vi "Vision Processing.vi"(4 "error in (no error)":errorcluster, 7 "Image Size":T1=enum."320x240") -> ()   [LabVIEW 2018]
doc: "This VI runs in parallel to other tasks. It gets images from the camera, processes them for color or shape and use that information to affect robot behavior."
uses:
  <vilib>/Rock Robotics/WPI/Camera/WPI_CameraImageSize.ctl
  <vilib>/Rock Robotics/WPI/Camera/WPI_CameraWhite Balance Values.ctl
  <vilib>/Rock Robotics/WPI/Camera/WPI_CameraExposure Values.ctl
  <vilib>/Rock Robotics/WPI/Camera/WPI_CameraFrameRate.ctl
  Robot Global Data.vi
panel:
  in  "Image Size 2":T1=enum."320x240"
  in  "error in (no error) 2":errorcluster
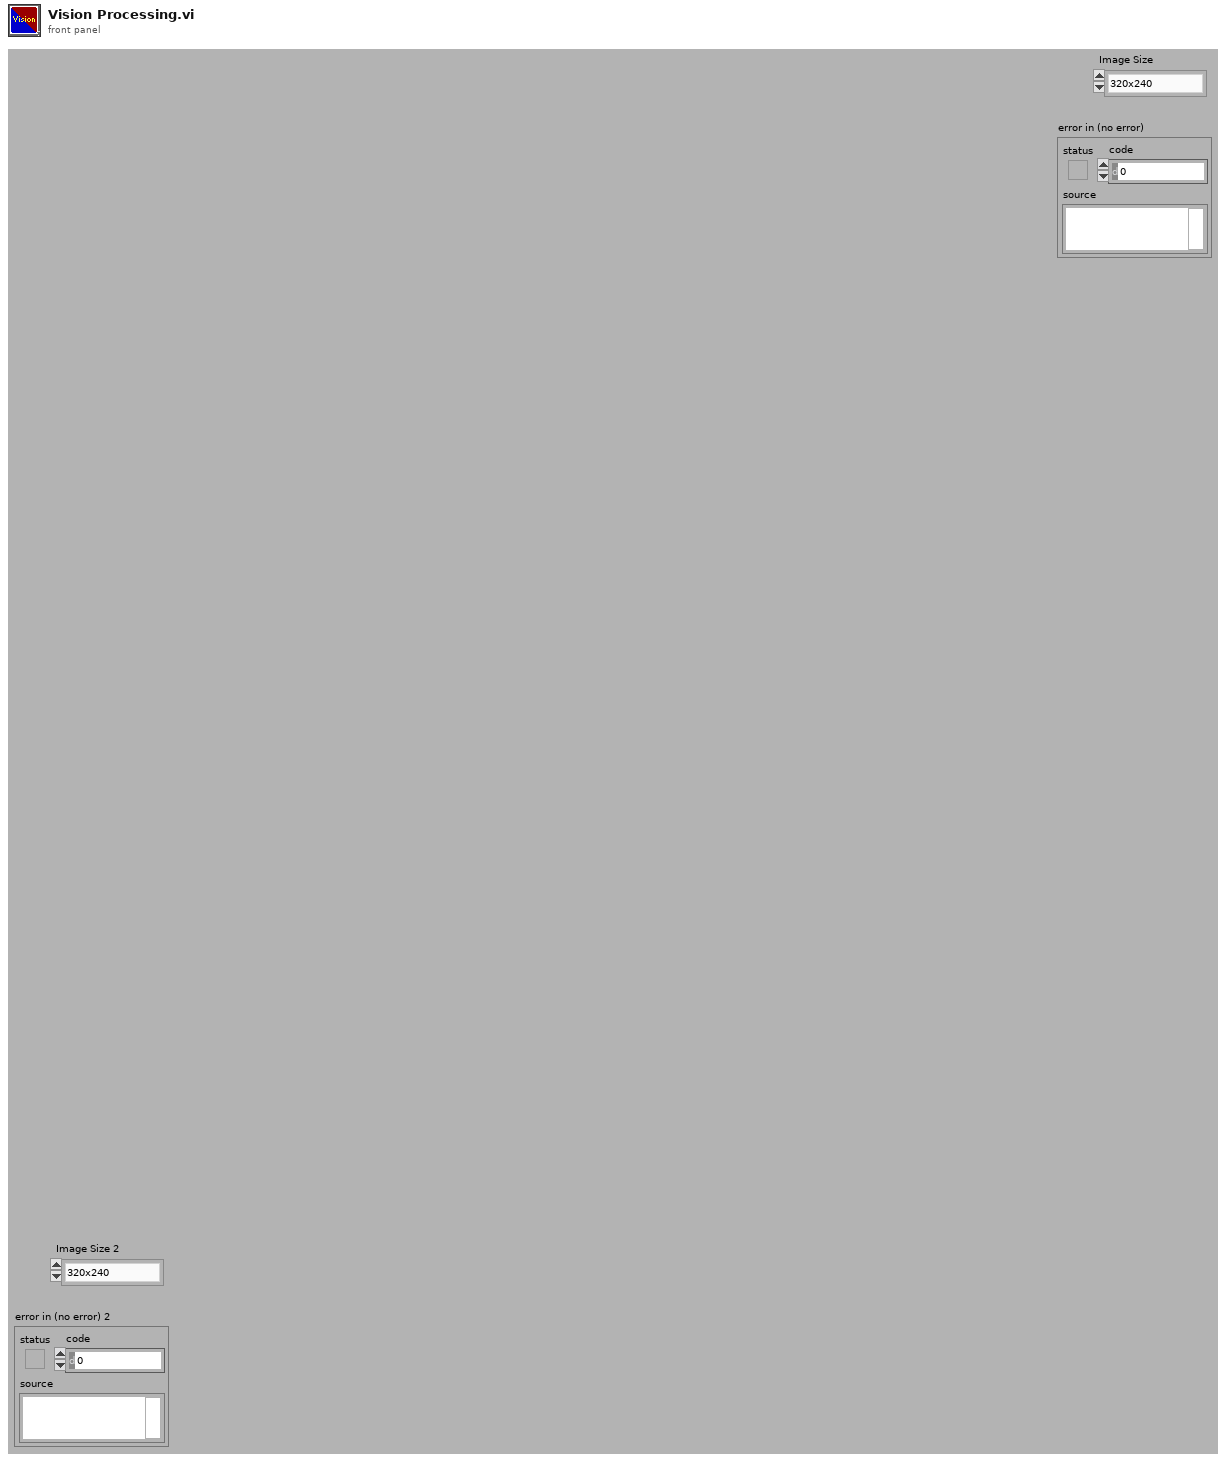
[diagram p1: front panel]
types:
  T1 = typedef "WPI_CameraImageSize.ctl" = enum16{"640x480", "320x240", "160x120", "Custom"}
  T2 = typedef "WPI_CameraFrameRate.ctl" = u32
  T3 = typedef "WPI_CameraExposure Values.ctl" = enum16{"Auto", "Flicker-free 50 Hz", "Flicker-free 60 Hz", "Hold current", "Custom"}
  T4 = typedef "WPI_CameraWhite Balance Values.ctl" = enum16{"Auto", "Fixed indoor", "Fixed outdoor 1", "Fixed outdoor 2", "Fixed fluorescent 1", "Fixed fluorescent 2", "Hold current", "Custom"}
  T5 = typedef "Image Type" = u32
  T6 = typedef "WPI_CameraDevRef.ctl" = cluster{"Camera Address":string, "CameraStatus":errorcluster}
  T7 = typedef "IMAQ Image.ctl" = refnum<image>
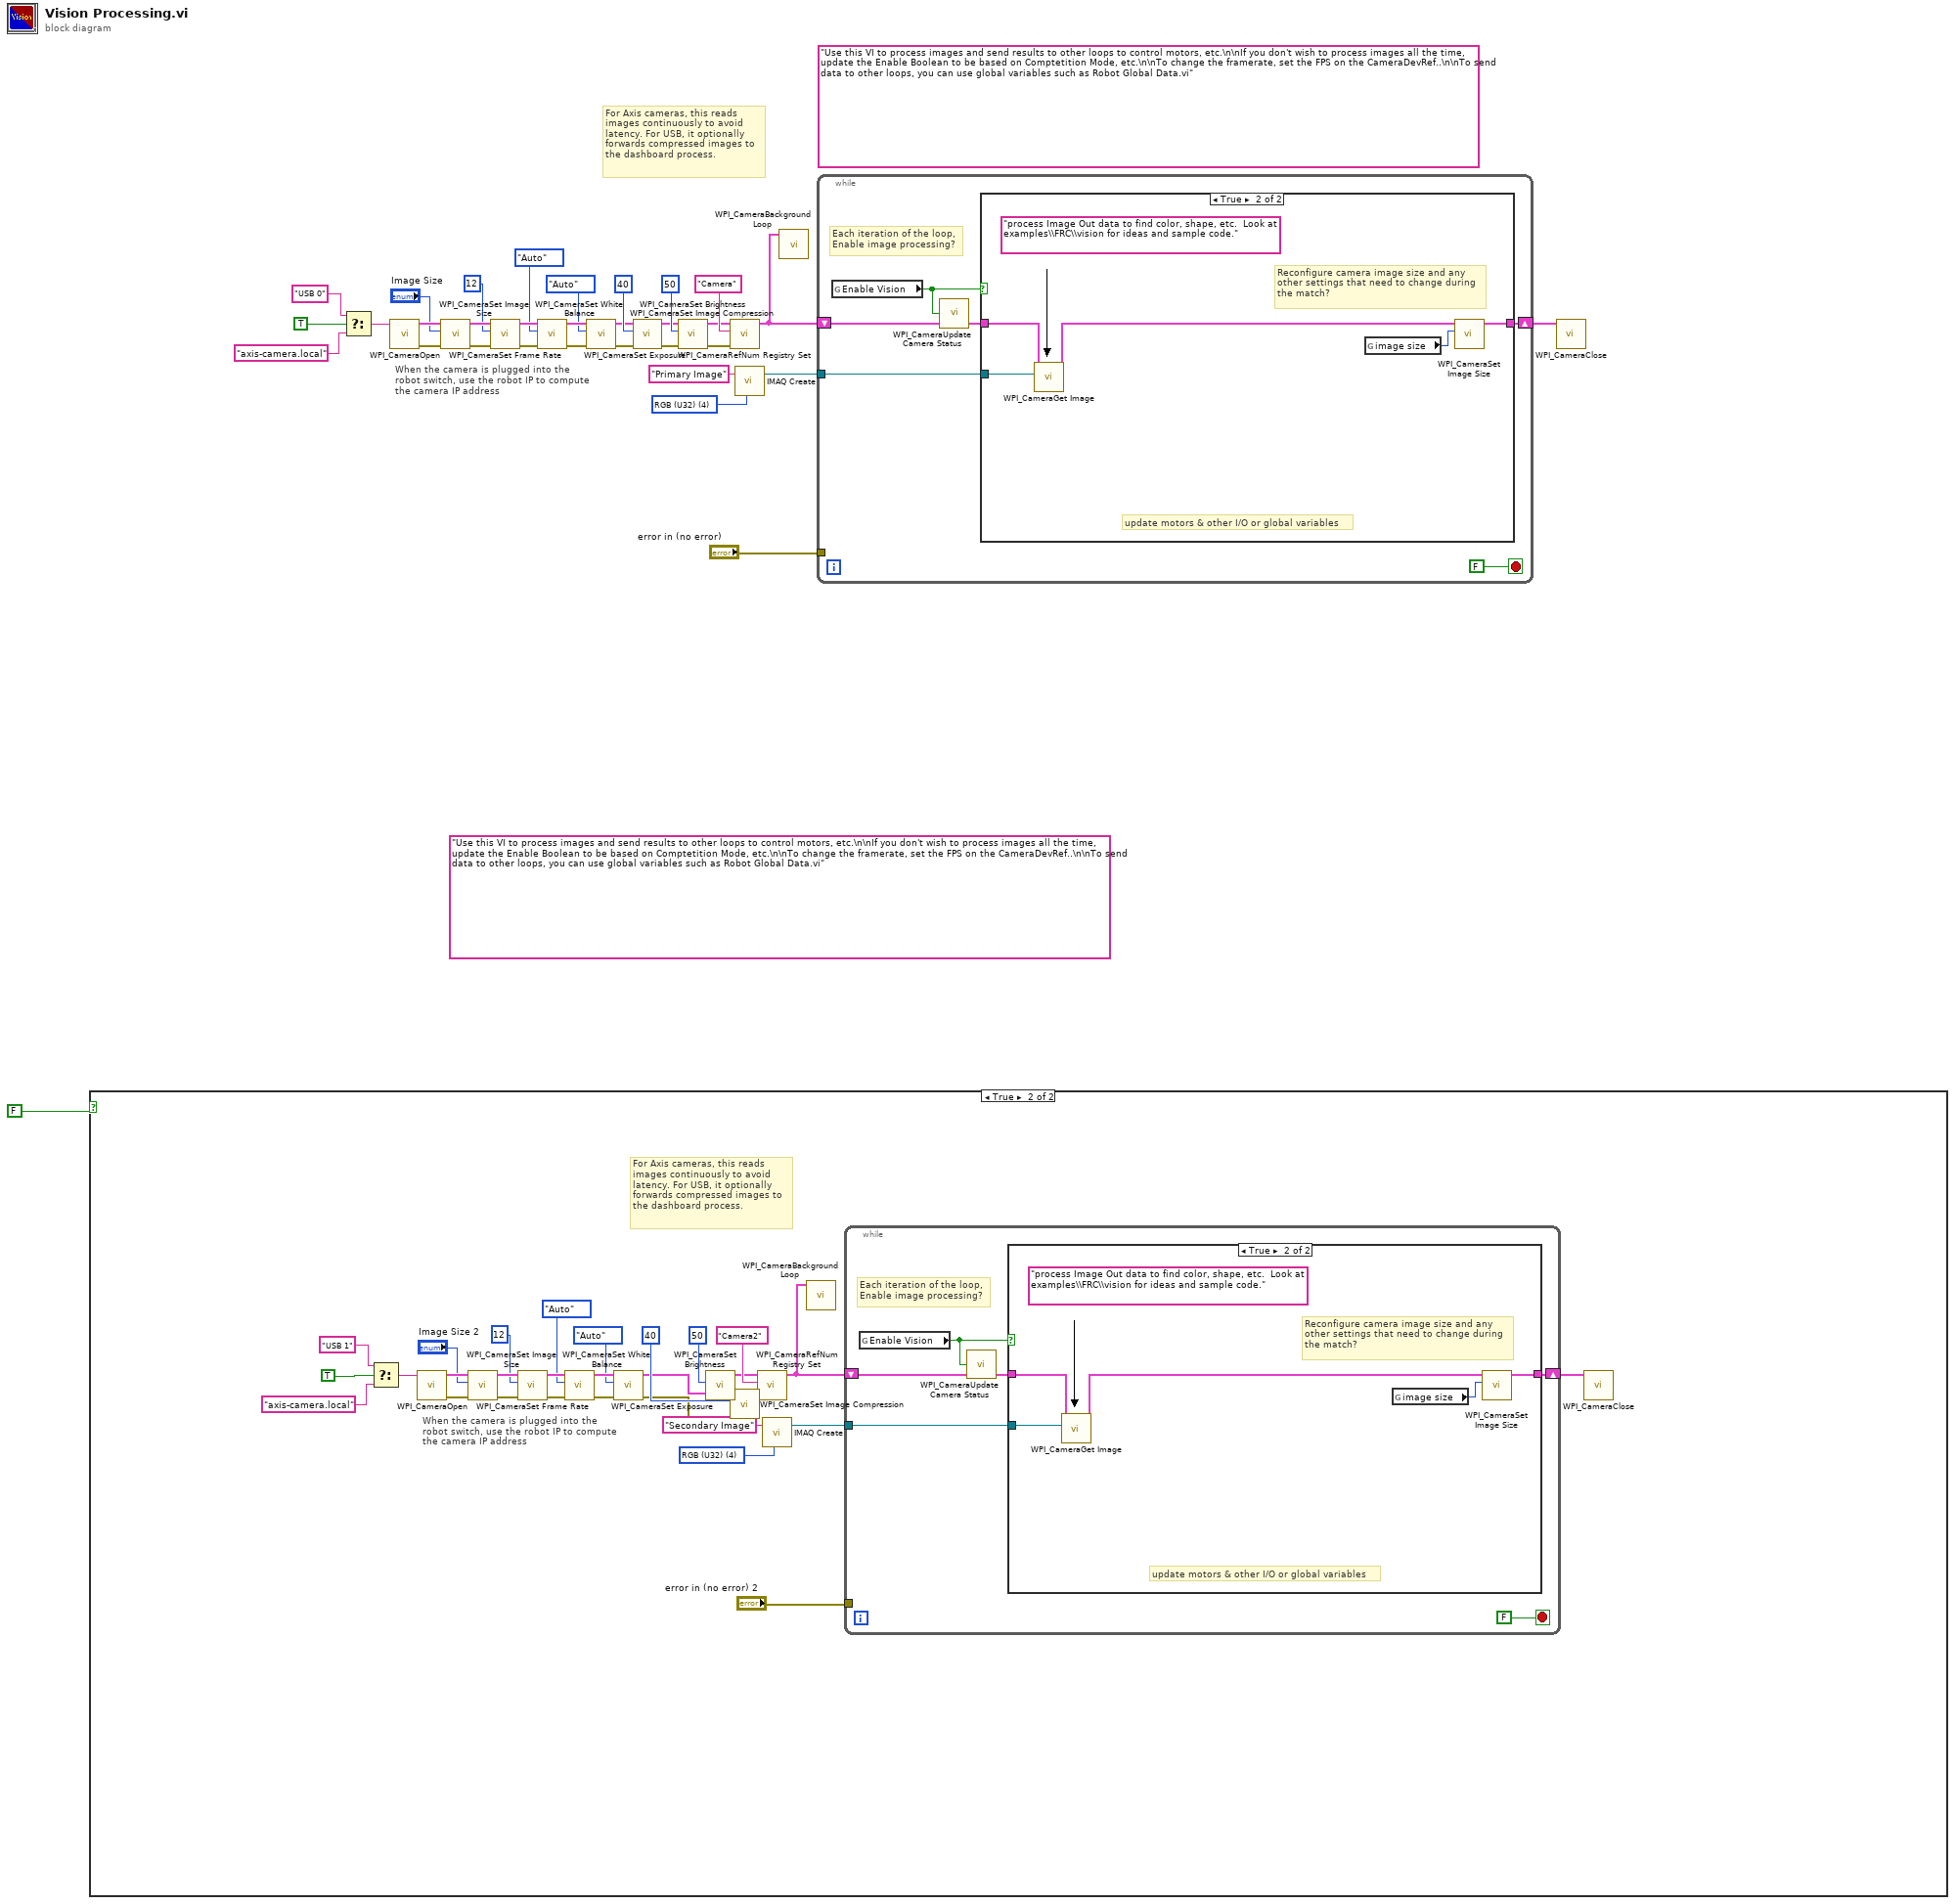
[diagram p0: block diagram]
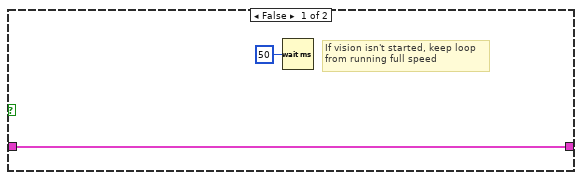
[diagram p3: hidden frame]
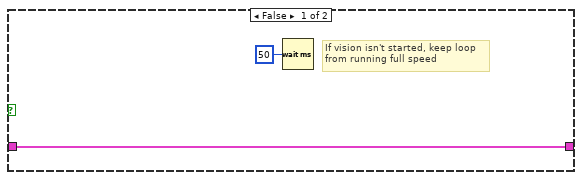
[diagram p4: hidden frame]
diagram:
  (unwired) "Use this VI to process images and send results to other loops to control motors, etc.\n\nIf you don't wish to process images all the time, update the Enable Boolean to be based on Comptetition Mode, etc.\n\nTo change the framerate, set the FPS on the CameraDevRef..\n\nTo send data to other loops, you can use global variables such as Robot Global Data.vi"
  (unwired) "Use this VI to process images and send results to other loops to control motors, etc.\n\nIf you don't wish to process images all the time, update the Enable Boolean to be based on Comptetition Mode, etc.\n\nTo change the framerate, set the FPS on the CameraDevRef..\n\nTo send data to other loops, you can use global variables such as Robot Global Data.vi"
  w32 = T5 4 items=["Grayscale (U8)", "Grayscale (I16)", "Grayscale (SGL)", "Complex (CSG)", "RGB (U32)", "HSL (U32)", "RGB (U64)"] ("Image Type")
  # "When the camera is plugged into the\nrobot switch, use the robot IP to compute\nthe camera IP address"
  # "For Axis cameras, this reads\nimages continuously to avoid\nlatency. For USB, it optionally\nforwards compressed images to\nthe dashboard process."
  n1 = case shown="True" FALSE {
    frame False {
    }
    frame True {
      w63 = T5 4 items=["Grayscale (U8)", "Grayscale (I16)", "Grayscale (SGL)", "Complex (CSG)", "RGB (U32)", "HSL (U32)", "RGB (U64)"] ("Image Type")
      # "When the camera is plugged into the\nrobot switch, use the robot IP to compute\nthe camera IP address"
      # "For Axis cameras, this reads\nimages continuously to avoid\nlatency. For USB, it optionally\nforwards compressed images to\nthe dashboard process."
      n2 = Select(t="USB 1" ("format string"), s=TRUE ("dot notation? (F)"), f="axis-camera.local" ("format string")) -> (s? t:f=w34:string)
      n3 = call <vilib>:"WPI_CameraOpen.vi"("Camera Address"=w34) -> ("error out"=w51:errorcluster, "CameraDevRef"=w52:T6)  [unwired: 1 in, 8 out]
      n4 = call <vilib>:"WPI_CameraSet Image Size.vi"("error in (no error)"=w51, "Image Size"="Image Size 2", "CameraDevRef"=w52) -> ("error out"=w50:errorcluster, "CameraDevRef Out"=w53:T6)  [unwired: 1 in, 6 out]
      n5 = call <vilib>:"WPI_CameraSet Frame Rate.vi"("error in (no error)"=w50, "Frame Rate (fps)"=T2 12, "CameraDevRef"=w53) -> ("error out"=w49:errorcluster, "CameraDevRef Out"=w55:T6)  [unwired: 7 out]
      n6 = call <vilib>:"WPI_CameraSet White Balance.vi"("error in (no error)"=w49, "White Balance"=WPI_CameraWhite_Balance_Values."Auto", "CameraDevRef"=w55) -> ("error out"=w48:errorcluster, "CameraDevRef Out"=w54:T6)  [unwired: 1 in, 6 out]
      n7 = call <vilib>:"WPI_CameraSet Exposure.vi"("error in (no error)"=w48, "Exposure"=WPI_CameraExposure_Values."Auto", "CameraDevRef"=w54) -> ("error out"=w47:errorcluster, "CameraDevRef Out"=w57:T6)  [unwired: 1 in, 6 out]
      n8 = call <vilib>:"WPI_CameraSet Image Compression.vi"("error in (no error)"=w47, "Compression"=40, "CameraDevRef"=w57) -> ("error out"=w46:errorcluster, "CameraDevRef Out"=w56:T6)  [unwired: 7 out]
      n9 = call <vilib>:"WPI_CameraSet Brightness.vi"("error in (no error)"=w46, "Brightness"=50, "CameraDevRef"=w56) -> ("error out"=w44:errorcluster, "CameraDevRef Out"=w45:T6)  [unwired: 1 in, 6 out]
      n10 = call <vilib>:"WPI_CameraRefNum Registry Set.vi"("error in (no error)"=w44, "refnum name"="Camera2", "CameraDevRef"=w45) -> ("CameraDevRef"=w40:T6)  [unwired: 1 in, 7 out]
      n11 = call "IMAQ Create"("Image Name"="Secondary Image", "Image Type"=w63) -> ("New Image"=w61:T7)  [unwired: 2 in, 2 out]
      n12 = call <vilib>:"WPI_CameraBackground Loop.vi"("CameraDevRef"=w40) -> ()  [unwired: 11 in]
      n13 = while {
        shift-right: [w68] -> w38
        shift-left: w40 -> [w66]
        tunnel: w61 -> [w67]
        tunnel: "error in (no error) 2" -> [_]
        stop <- FALSE stop-if-true
        # "Each iteration of the loop,\nEnable image processing?"
        n14 = global read "Robot Global Data.vi" "Enable Vision"() -> (w64:bool)
        n15 = call <vilib>:"WPI_CameraUpdate Camera Status.vi"("CameraDevRef In"=w66, "Enable Vision"=w64) -> ("CameraDevRef Out"=w65:T6)  [unwired: 3 in]
        n16 = case shown="True" w64 {
          tunnel: w67 -> [_ w75]
          tunnel: [w71 w76] -> w68
          tunnel: w65 -> [w71 w73]
          frame False {
            # "If vision isn't started, keep loop\nfrom running full speed"
            n17 = Wait (ms)(milliseconds to wait=u32 50) -> ()  [unwired: 1 out]
          }
          frame True {
            (unwired) "process Image Out data to find color, shape, etc.  Look at examples\\FRC\\vision for ideas and sample code."
            # "update motors & other I/O or global variables"
            # "Reconfigure camera image size and any\nother settings that need to change during\nthe match?"
            n18 = call <vilib>:"WPI_CameraGet Image.vi"("Image"=w75, "CameraDevRef"=w73) -> ("CameraDevRef Out"=w72:T6)  [unwired: 1 in, 8 out]
            n19 = global read "Robot Global Data.vi" "image size"() -> (w74:T1)
            n20 = call <vilib>:"WPI_CameraSet Image Size.vi"("Image Size"=w74, "CameraDevRef"=w72) -> ("CameraDevRef Out"=w76:T6)  [unwired: 2 in, 7 out]
          }
        }
      }
      n21 = call <vilib>:"WPI_CameraClose.vi"("CameraDevRef"=w38) -> ()  [unwired: 1 in, 10 out]
    }
  }
  n22 = Select(t="USB 0" ("format string"), s=TRUE ("dot notation? (F)"), f="axis-camera.local" ("format string")) -> (s? t:f=w3:string)
  n23 = call <vilib>:"WPI_CameraOpen.vi"("Camera Address"=w3) -> ("error out"=w20:errorcluster, "CameraDevRef"=w21:T6)  [unwired: 1 in, 8 out]
  n24 = call <vilib>:"WPI_CameraSet Image Size.vi"("error in (no error)"=w20, "Image Size"="Image Size", "CameraDevRef"=w21) -> ("error out"=w19:errorcluster, "CameraDevRef Out"=w22:T6)  [unwired: 1 in, 6 out]
  n25 = call <vilib>:"WPI_CameraSet Frame Rate.vi"("error in (no error)"=w19, "Frame Rate (fps)"=T2 12, "CameraDevRef"=w22) -> ("error out"=w18:errorcluster, "CameraDevRef Out"=w24:T6)  [unwired: 7 out]
  n26 = call <vilib>:"WPI_CameraSet White Balance.vi"("error in (no error)"=w18, "White Balance"=WPI_CameraWhite_Balance_Values."Auto", "CameraDevRef"=w24) -> ("error out"=w17:errorcluster, "CameraDevRef Out"=w23:T6)  [unwired: 1 in, 6 out]
  n27 = call <vilib>:"WPI_CameraSet Exposure.vi"("error in (no error)"=w17, "Exposure"=WPI_CameraExposure_Values."Auto", "CameraDevRef"=w23) -> ("error out"=w16:errorcluster, "CameraDevRef Out"=w26:T6)  [unwired: 1 in, 6 out]
  n28 = call <vilib>:"WPI_CameraSet Image Compression.vi"("error in (no error)"=w16, "Compression"=40, "CameraDevRef"=w26) -> ("error out"=w15:errorcluster, "CameraDevRef Out"=w25:T6)  [unwired: 7 out]
  n29 = call <vilib>:"WPI_CameraSet Brightness.vi"("error in (no error)"=w15, "Brightness"=50, "CameraDevRef"=w25) -> ("error out"=w13:errorcluster, "CameraDevRef Out"=w14:T6)  [unwired: 1 in, 6 out]
  n30 = call <vilib>:"WPI_CameraRefNum Registry Set.vi"("error in (no error)"=w13, "refnum name"="Camera", "CameraDevRef"=w14) -> ("CameraDevRef"=w9:T6)  [unwired: 1 in, 7 out]
  n31 = call "IMAQ Create"("Image Name"="Primary Image", "Image Type"=w32) -> ("New Image"=w30:T7)  [unwired: 2 in, 2 out]
  n32 = call <vilib>:"WPI_CameraBackground Loop.vi"("CameraDevRef"=w9) -> ()  [unwired: 11 in]
  n33 = while {
    shift-right: [w81] -> w7
    shift-left: w9 -> [w79]
    tunnel: w30 -> [w80]
    tunnel: "error in (no error)" -> [_]
    stop <- FALSE stop-if-true
    # "Each iteration of the loop,\nEnable image processing?"
    n34 = global read "Robot Global Data.vi" "Enable Vision"() -> (w77:bool)
    n35 = call <vilib>:"WPI_CameraUpdate Camera Status.vi"("CameraDevRef In"=w79, "Enable Vision"=w77) -> ("CameraDevRef Out"=w78:T6)  [unwired: 3 in]
    n36 = case shown="True" w77 {
      tunnel: w80 -> [_ w88]
      tunnel: [w84 w89] -> w81
      tunnel: w78 -> [w84 w86]
      frame False {
        # "If vision isn't started, keep loop\nfrom running full speed"
        n37 = Wait (ms)(milliseconds to wait=u32 50) -> ()  [unwired: 1 out]
      }
      frame True {
        (unwired) "process Image Out data to find color, shape, etc.  Look at examples\\FRC\\vision for ideas and sample code."
        # "update motors & other I/O or global variables"
        # "Reconfigure camera image size and any\nother settings that need to change during\nthe match?"
        n38 = call <vilib>:"WPI_CameraGet Image.vi"("Image"=w88, "CameraDevRef"=w86) -> ("CameraDevRef Out"=w85:T6)  [unwired: 1 in, 8 out]
        n39 = global read "Robot Global Data.vi" "image size"() -> (w87:T1)
        n40 = call <vilib>:"WPI_CameraSet Image Size.vi"("Image Size"=w87, "CameraDevRef"=w85) -> ("CameraDevRef Out"=w89:T6)  [unwired: 2 in, 7 out]
      }
    }
  }
  n41 = call <vilib>:"WPI_CameraClose.vi"("CameraDevRef"=w7) -> ()  [unwired: 1 in, 10 out]
